vi "FSM.vi"() -> ()   [LabVIEW 2015]
uses:
  states.ctl
  globals.vi
  <vilib>/Utility/file.llb/Read Delimited Spreadsheet (DBL).vi
  read_file.vi
  output_byte.vi
panel:
  out "Progress":dbl(slide) scale=0.0..100.0
  out "Angle accuracy":dbl
  out "Current shoulder angle":dbl
  out "Current elbow angle":dbl
  in  "Stop":bool
  out "Desired shoulder Angle":dbl
  out "Desired elbow Angle":dbl
  out "Number of rows":dbl
  out "Row number":dbl
  in  "Start Button":bool
  out "State to Recover from":T1
  out "Current State":T1
  in  "Pause":bool
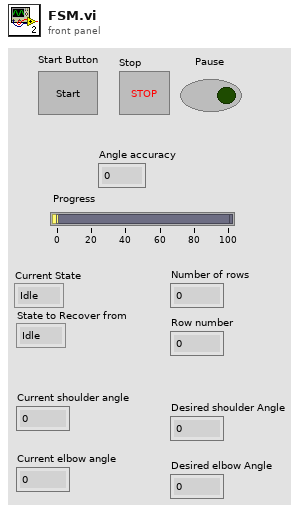
[diagram p1: front panel]
types:
  T1 = typedef "states.ctl" = enum16{"Idle", "Pause", "Next Contour", "Aligning", "Lowering Pen", "Drawing", "Next Point", "Lifting Pen", "Stop", "Put Away"}
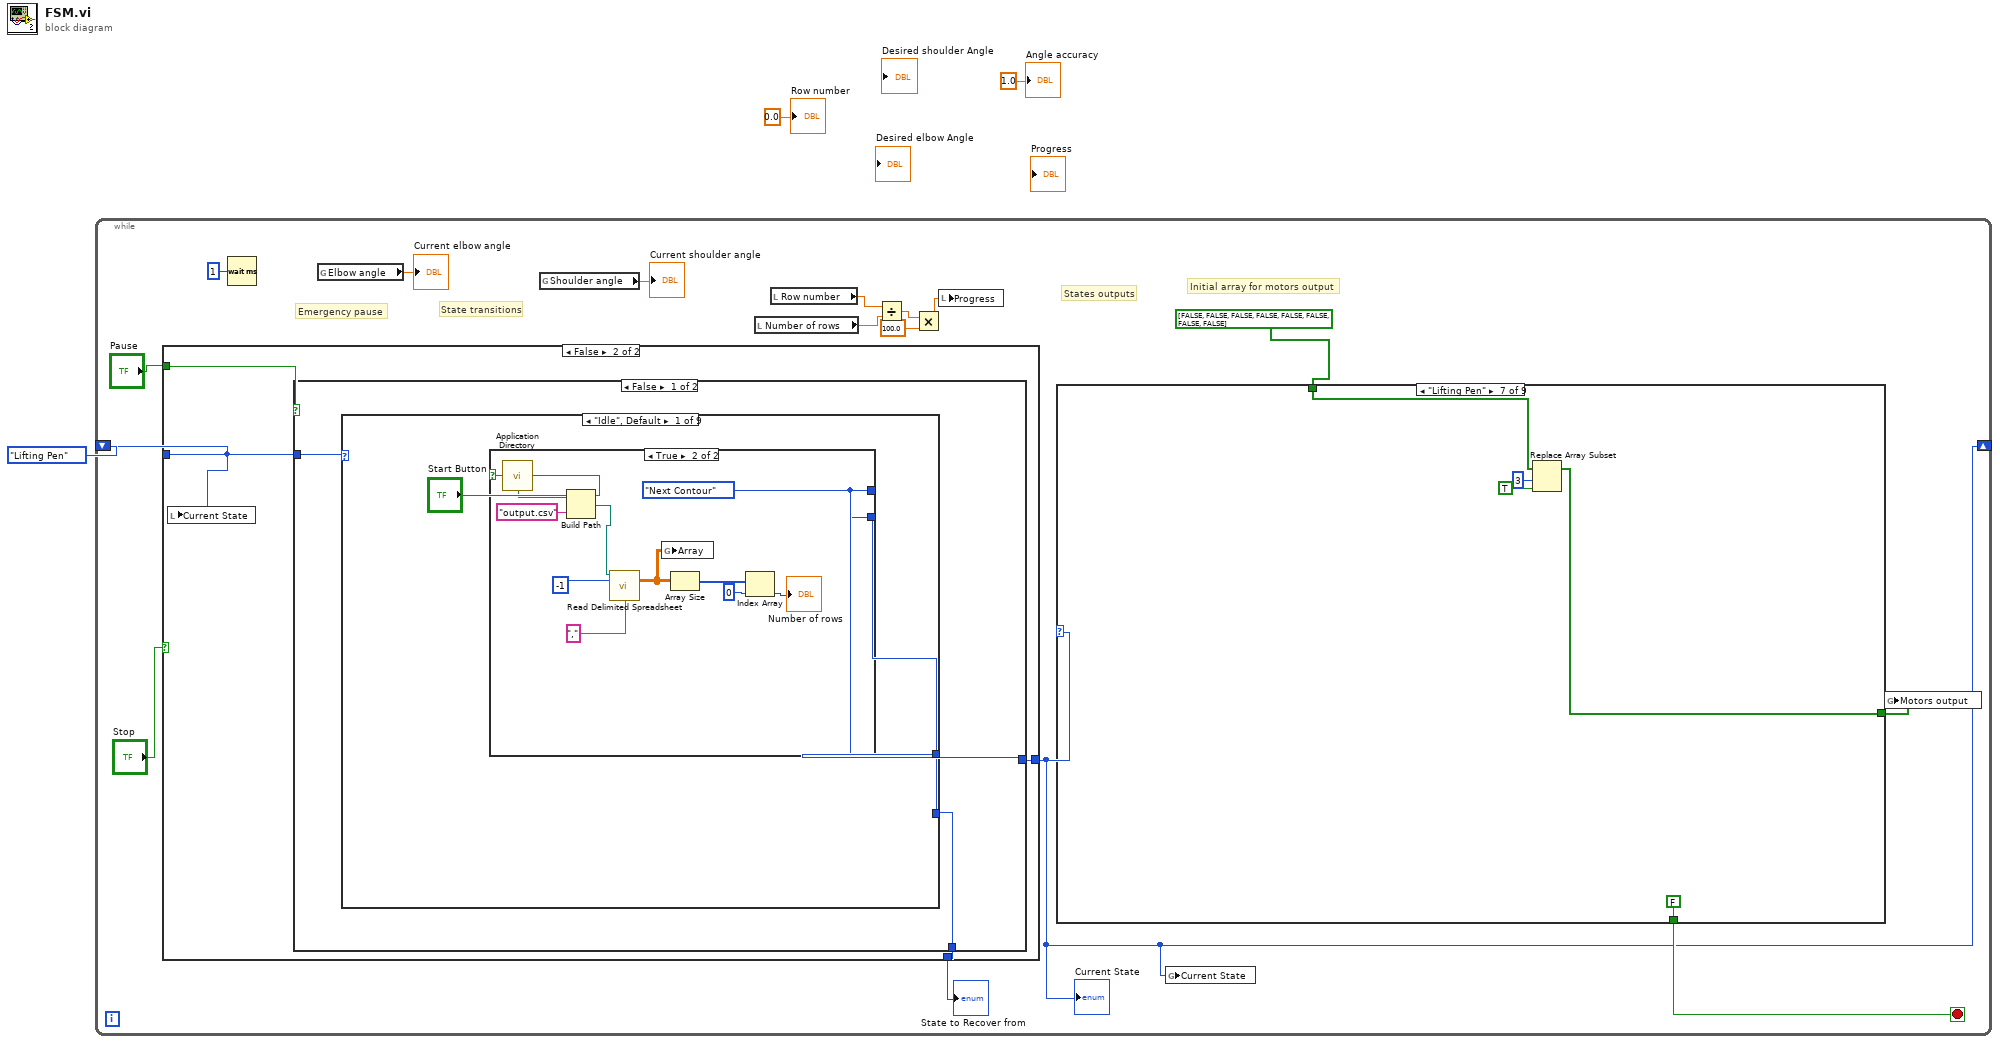
[diagram p0: block diagram]
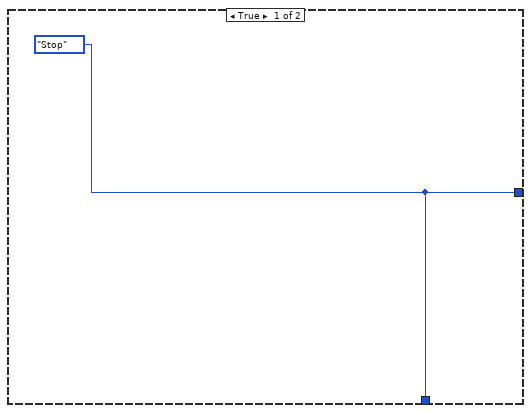
[diagram p2: hidden frame]
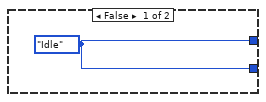
[diagram p3: hidden frame]
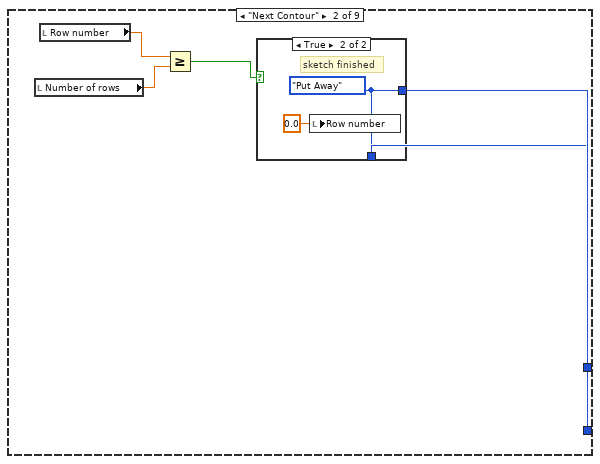
[diagram p4: hidden frame]
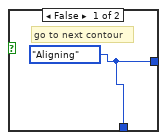
[diagram p5: hidden frame]
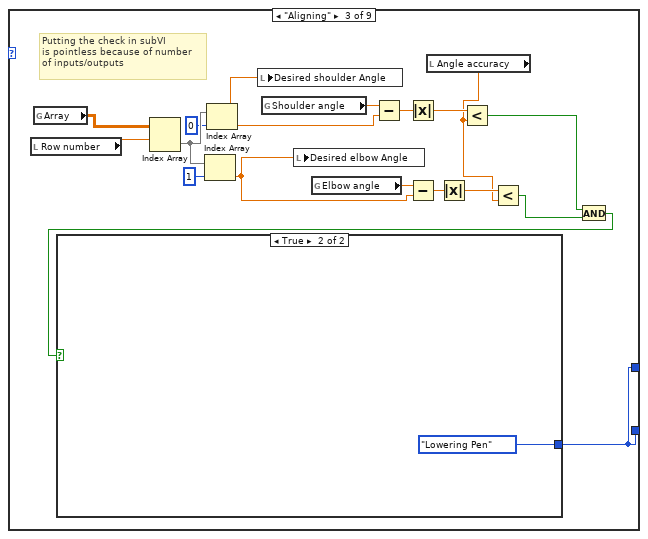
[diagram p6: hidden frame]
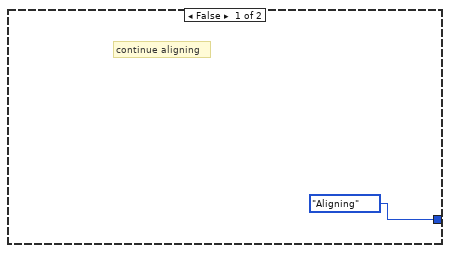
[diagram p7: hidden frame]
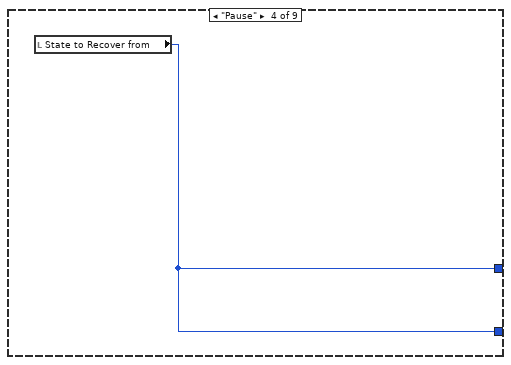
[diagram p8: hidden frame]
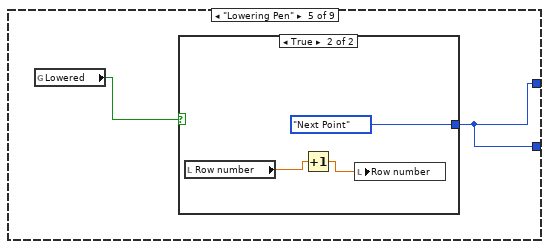
[diagram p9: hidden frame]
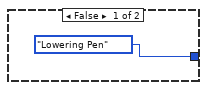
[diagram p10: hidden frame]
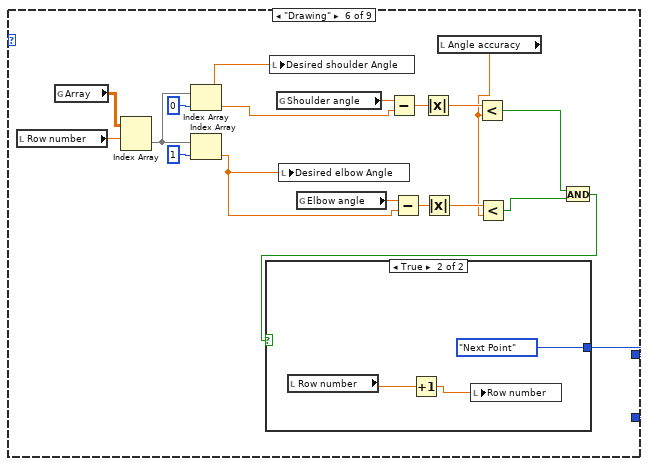
[diagram p11: hidden frame]
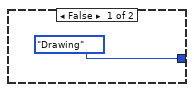
[diagram p12: hidden frame]
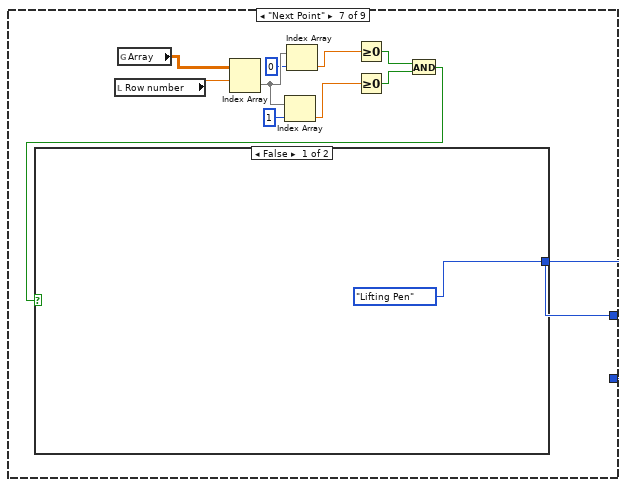
[diagram p13: hidden frame]
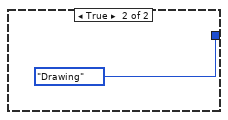
[diagram p14: hidden frame]
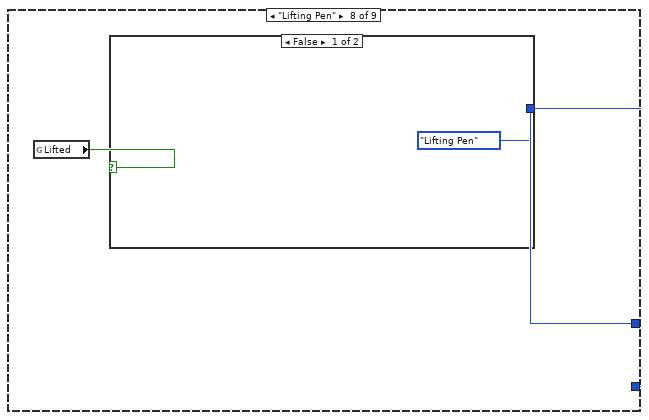
[diagram p15: hidden frame]
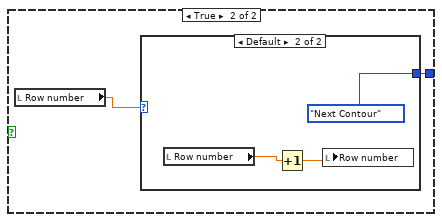
[diagram p16: hidden frame]
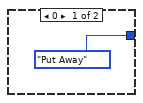
[diagram p17: hidden frame]
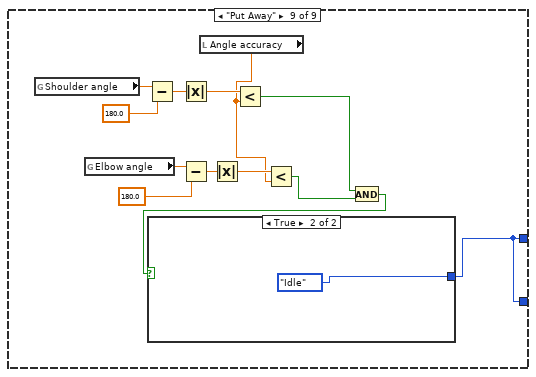
[diagram p18: hidden frame]
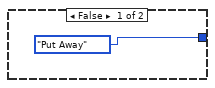
[diagram p19: hidden frame]
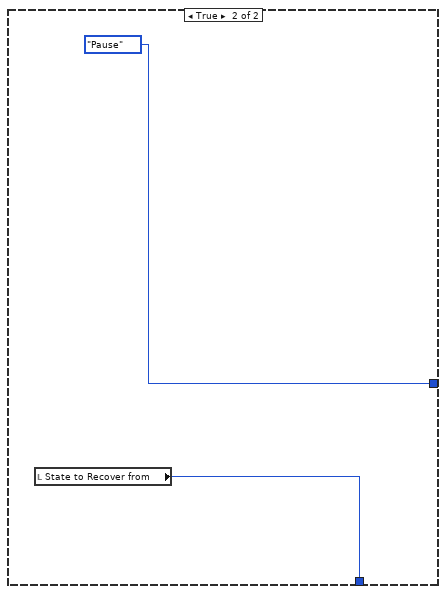
[diagram p20: hidden frame]
diagram:
  n1 = while {
    shift-right: [w4] -> _
    shift-left: states."Lifting Pen" ("State") -> [w18]
    stop <- w5 stop-if-true
    # "Initial array for motors output"
    # "States outputs"
    # "State transitions"
    # "Emergency pause"
    n2 = case shown="False" "Stop" {
      tunnel: "Pause" -> [_ w24]
      tunnel: w18 -> [_ w23]
      tunnel: [w20 w22] -> w14
      tunnel: [w20 w21] -> w4
      frame True {
        w20 = states."Stop" ("State")
      }
      frame False {
        n3 = local write "Current State"(w23) -> ()
        n4 = case shown="False" w24 {
          tunnel: w23 -> [w27 _]
          tunnel: [w26 states."Pause" ("State")] -> w21
          tunnel: [w25 w136] -> w22
          frame False {
            n5 = case shown="\"Idle\", Default" w27 {
              tunnel: [w29 w46 w54 w70 w72 w80 w100 w113 w121] -> w26
              tunnel: [w28 w45 w54 w70 w72 w80 w100 w113 w121] -> w25
              frame "Idle", Default {
                n6 = case shown="True" "Start Button" {
                  tunnel: [w31 w41] -> w29
                  tunnel: [w31 w41] -> w28
                  frame False {
                    w31 = states."Idle" ("State")
                  }
                  frame True {
                    w41 = states."Next Contour" ("State")
                    n7 = call <vilib>:"Application Directory.vi"() -> ("Application Directory"=w33:path)
                    n8 = Build Path(base path=w33, name or relative path="output.csv") -> (appended path=w32:path)
                    n9 = call-poly <vilib>:"Read Delimited Spreadsheet.vi"("file path (dialog if empty)"=w32, "number of rows (all:-1)"=-1, "delimiter (\\t)"="," ("delimiter (\\t)")) -> ("all rows"=w40:dbl[][])  [unwired: 7 in, 5 out]
                    n10 = global write "read_file.vi" "Array"(w40) -> ()
                    n11 = Array Size(array=w40) -> (size(s)=w36:i32[])
                    n12 = Index Array(array=w36, index=0) -> (element=→"Number of rows":i32)
                  }
                }
              }
              frame "Next Contour" {
                n13 = local read "Number of rows"() -> (w43:dbl)
                n14 = local read "Row number"() -> (w44:dbl)
                n15 = Greater Or Equal?(x=w44, y=w43) -> (x >= y?=w42:bool)
                n16 = case shown="True" w42 {
                  tunnel: [w47 w49] -> w46
                  tunnel: [w47 w49] -> w45
                  frame False {
                    w47 = states."Aligning" ("State")
                    # "go to next contour"
                  }
                  frame True {
                    w49 = states."Put Away" ("State")
                    # "sketch finished"
                    n17 = local write "Row number"(0.0 ("Row number")) -> ()
                  }
                }
              }
              frame "Aligning" {
                # "Putting the check in subVI\nis pointless because of number\nof inputs/outputs"
                n18 = local read "Row number"() -> (w66:dbl)
                n19 = global read "read_file.vi" "Array"() -> (w67:dbl[][])
                n20 = Index Array(array=w67, index (row)=w66) -> (element=w65:dbl[])  [unwired: 1 in]
                n21 = Index Array(array=w65, index=1) -> (element=w57:dbl)
                n22 = Index Array(array=w65, index=0) -> (element=w58:dbl)
                n23 = local write "Desired shoulder Angle"(w58) -> ()
                n24 = global read "globals.vi" "Shoulder angle"() -> (w53:dbl)
                n25 = local write "Desired elbow Angle"(w57) -> ()
                n26 = global read "globals.vi" "Elbow angle"() -> (w52:dbl)
                n27 = Subtract(x=w53, y=w58) -> (x-y=w62:dbl)
                n28 = Absolute Value(x=w62) -> (abs(x)=w61:dbl)
                n29 = Subtract(x=w52, y=w57) -> (x-y=w60:dbl)
                n30 = local read "Angle accuracy"() -> (w50:dbl)
                n31 = Absolute Value(x=w60) -> (abs(x)=w59:dbl)
                n32 = Less?(x=w61, y=w50) -> (x < y?=w56:bool)
                n33 = Less?(x=w59, y=w50) -> (x < y?=w55:bool)
                n34 = And(x=w56, y=w55) -> (x .and. y?=w51:bool)
                n35 = case shown="True" w51 {
                  tunnel: [states."Aligning" ("State") states."Lowering Pen" ("State")] -> w54
                  frame False {
                    # "continue aligning"
                  }
                  frame True {
                  }
                }
              }
              frame "Pause" {
                n36 = local read "State to Recover from"() -> (w70:T1)
              }
              frame "Lowering Pen" {
                n37 = global read "globals.vi" "Lowered"() -> (w71:bool)
                n38 = case shown="True" w71 {
                  tunnel: [states."Lowering Pen" ("State") states."Next Point" ("State")] -> w72
                  frame False {
                  }
                  frame True {
                    n39 = local read "Row number"() -> (w74:dbl)
                    n40 = Increment(x=w74) -> (x+1=w75:dbl)
                    n41 = local write "Row number"(w75) -> ()
                  }
                }
              }
              frame "Drawing" {
                n42 = local read "Row number"() -> (w81:dbl)
                n43 = global read "read_file.vi" "Array"() -> (w94:dbl[][])
                n44 = Index Array(array=w94, index (row)=w81) -> (element=w93:dbl[])  [unwired: 1 in]
                n45 = Index Array(array=w93, index=0) -> (element=w79:dbl)
                n46 = Index Array(array=w93, index=1) -> (element=w86:dbl)
                n47 = local write "Desired shoulder Angle"(w79) -> ()
                n48 = global read "globals.vi" "Shoulder angle"() -> (w83:dbl)
                n49 = local write "Desired elbow Angle"(w86) -> ()
                n50 = global read "globals.vi" "Elbow angle"() -> (w82:dbl)
                n51 = Subtract(x=w83, y=w79) -> (x-y=w90:dbl)
                n52 = Subtract(x=w82, y=w86) -> (x-y=w88:dbl)
                n53 = Absolute Value(x=w90) -> (abs(x)=w89:dbl)
                n54 = Absolute Value(x=w88) -> (abs(x)=w87:dbl)
                n55 = local read "Angle accuracy"() -> (w77:dbl)
                n56 = Less?(x=w89, y=w77) -> (x < y?=w85:bool)
                n57 = Less?(x=w87, y=w77) -> (x < y?=w84:bool)
                n58 = And(x=w85, y=w84) -> (x .and. y?=w78:bool)
                n59 = case shown="True" w78 {
                  tunnel: [states."Drawing" ("State") states."Next Point" ("State")] -> w80
                  frame False {
                  }
                  frame True {
                    n60 = local read "Row number"() -> (w97:dbl)
                    n61 = Increment(x=w97) -> (x+1=w96:dbl)
                    n62 = local write "Row number"(w96) -> ()
                  }
                }
              }
              frame "Next Point" {
                n63 = local read "Row number"() -> (w108:dbl)
                n64 = global read "read_file.vi" "Array"() -> (w109:dbl[][])
                n65 = Index Array(array=w109, index (row)=w108) -> (element=w107:dbl[])  [unwired: 1 in]
                n66 = Index Array(array=w107, index=1) -> (element=w103:dbl)
                n67 = Index Array(array=w107, index=0) -> (element=w104:dbl)
                n68 = Greater Or Equal To 0?(x=w104) -> (x >= 0?=w102:bool)
                n69 = Greater Or Equal To 0?(x=w103) -> (x >= 0?=w101:bool)
                n70 = And(x=w102, y=w101) -> (x .and. y?=w99:bool)
                n71 = case shown="False" w99 {
                  tunnel: [states."Lifting Pen" ("State") states."Drawing" ("State")] -> w100
                  frame False {
                  }
                  frame True {
                  }
                }
              }
              frame "Lifting Pen" {
                n72 = global read "globals.vi" "Lifted"() -> (w112:bool)
                n73 = case shown="False" w112 {
                  tunnel: [states."Lifting Pen" ("State") w116] -> w113
                  frame False {
                  }
                  frame True {
                    n74 = local read "Row number"() -> (w115:dbl)
                    n75 = case shown="Default" w115 {
                      tunnel: [states."Put Away" ("State") states."Next Contour" ("State")] -> w116
                      frame 0 {
                      }
                      frame Default {
                        n76 = local read "Row number"() -> (w119:dbl)
                        n77 = Increment(x=w119) -> (x+1=w118:dbl)
                        n78 = local write "Row number"(w118) -> ()
                      }
                    }
                  }
                }
              }
              frame "Put Away" {
                n79 = global read "globals.vi" "Shoulder angle"() -> (w127:dbl)
                n80 = global read "globals.vi" "Elbow angle"() -> (w126:dbl)
                n81 = Subtract(x=w127, y=180.0) -> (x-y=w133:dbl)
                n82 = Absolute Value(x=w133) -> (abs(x)=w132:dbl)
                n83 = Subtract(x=w126, y=180.0) -> (x-y=w131:dbl)
                n84 = local read "Angle accuracy"() -> (w125:dbl)
                n85 = Absolute Value(x=w131) -> (abs(x)=w130:dbl)
                n86 = Less?(x=w132, y=w125) -> (x < y?=w129:bool)
                n87 = Less?(x=w130, y=w125) -> (x < y?=w128:bool)
                n88 = And(x=w129, y=w128) -> (x .and. y?=w122:bool)
                n89 = case shown="True" w122 {
                  tunnel: [states."Put Away" ("State") states."Idle" ("State")] -> w121
                  frame False {
                  }
                  frame True {
                  }
                }
              }
            }
          }
          frame True {
            n90 = local read "State to Recover from"() -> (w136:T1)
          }
        }
      }
    }
    "Current State" <- w4
    "State to Recover from" <- w14
    n91 = Wait (ms)(milliseconds to wait=u32 1 ("millisecond multiple")) -> ()  [unwired: 1 out]
    n92 = global read "globals.vi" "Elbow angle"() -> (→"Current elbow angle":dbl)
    n93 = global read "globals.vi" "Shoulder angle"() -> (→"Current shoulder angle":dbl)
    n94 = local read "Number of rows"() -> (w10:dbl)
    n95 = local read "Row number"() -> (w11:dbl)
    n96 = Divide(x=w11, y=w10) -> (x/y=w9:dbl)
    n97 = Multiply(x=w9, y=100.0) -> (x*y=w7:dbl)
    n98 = local write "Progress"(w7) -> ()
    n99 = case shown="\"Lifting Pen\"" w4 {
      tunnel: bool[] [FALSE, FALSE, FALSE, FALSE, FALSE, FALSE, FALSE, FALSE] -> [w139 w141 w143 w146 w167 w198 w201 w205 w209]
      tunnel: [w139 w141 w143 w145 w166 w198 w200 w205 w206] -> w12
      tunnel: [FALSE FALSE FALSE FALSE FALSE FALSE FALSE TRUE FALSE] -> w5
      frame "Idle", Default {
      }
      frame "Pause" {
      }
      frame "Next Contour" {
      }
      frame "Lowering Pen" {
        n100 = Replace Array Subset(array=w146, new element=TRUE ("new element/subarray"), index=2) -> (w145:bool[])
      }
      frame "Aligning", "Drawing" {
        n101 = local read "Row number"() -> (w162:dbl)
        n102 = global read "read_file.vi" "Array"() -> (w161:dbl[][])
        n103 = global read "globals.vi" "Shoulder angle"() -> (w160:dbl)
        n104 = global read "globals.vi" "Elbow angle"() -> (w156:dbl)
        n105 = Index Array(array=w161, index (row)=w162) -> (element=w163:dbl[])  [unwired: 1 in]
        n106 = Index Array(array=w163, index=1) -> (element=w153:dbl)
        n107 = local write "Desired elbow Angle"(w153) -> ()
        n108 = Index Array(array=w163, index=0) -> (element=w157:dbl)
        n109 = local write "Desired shoulder Angle"(w157) -> ()
        n110 = local read "Angle accuracy"() -> (w150:dbl)
        n111 = Subtract(x=w160, y=w157) -> (x-y=w158:dbl)
        n112 = Subtract(x=w156, y=w153) -> (x-y=w154:dbl)
        n113 = Absolute Value(x=w158) -> (abs(x)=w159:dbl)
        n114 = Absolute Value(x=w154) -> (abs(x)=w155:dbl)
        n115 = Less?(x=w159, y=w150) -> (x < y?=w152:bool)
        n116 = Less?(x=w155, y=w150) -> (x < y?=w151:bool)
        n117 = case shown="False" w151 {
          tunnel: [w184 w196] -> w168
          tunnel: w167 -> [w183 w196]
          frame False {
            n118 = local read "Desired elbow Angle"() -> (w187:dbl)
            n119 = global read "globals.vi" "Elbow angle"() -> (w185:dbl)
            n120 = Greater?(x=w185, y=w187) -> (0:w186:bool)
            n121 = case shown="False" w186 {
              tunnel: [w189 w193] -> w184
              tunnel: w183 -> [w188 w192]
              frame False {
                n122 = Replace Array Subset(array=w188, new element=TRUE ("new element/subarray"), index=5) -> (w189:bool[])
              }
              frame True {
                n123 = Replace Array Subset(array=w192, new element=TRUE ("new element/subarray"), index=4) -> (w193:bool[])
              }
            }
          }
          frame True {
          }
        }
        n124 = case shown="False" w152 {
          tunnel: [w171 w182] -> w166
          tunnel: w168 -> [w169 w182]
          frame False {
            n125 = local read "Desired shoulder Angle"() -> (w170:dbl)
            n126 = global read "globals.vi" "Shoulder angle"() -> (w172:dbl)
            n127 = Greater?(x=w172, y=w170) -> (0:w173:bool)
            n128 = case shown="False" w173 {
              tunnel: [w175 w179] -> w171
              tunnel: w169 -> [w174 w178]
              frame False {
                n129 = Replace Array Subset(array=w174, new element=TRUE ("new element/subarray"), index=7) -> (w175:bool[])
              }
              frame True {
                n130 = Replace Array Subset(array=w178, new element=TRUE ("new element/subarray"), index=6) -> (w179:bool[])
              }
            }
          }
          frame True {
          }
        }
      }
      frame "Next Point" {
      }
      frame "Lifting Pen" {
        n131 = Replace Array Subset(array=w201, new element=TRUE ("new element/subarray"), index=3) -> (w200:bool[])
      }
      frame "Stop" {
      }
      frame "Put Away" {
        n132 = global read "globals.vi" "Shoulder angle"() -> (w218:dbl)
        n133 = global read "globals.vi" "Elbow angle"() -> (w215:dbl)
        n134 = local read "Angle accuracy"() -> (w210:dbl)
        n135 = Subtract(x=w218, y=180.0) -> (x-y=w216:dbl)
        n136 = Subtract(x=w215, y=180.0) -> (x-y=w213:dbl)
        n137 = Absolute Value(x=w216) -> (abs(x)=w217:dbl)
        n138 = Absolute Value(x=w213) -> (abs(x)=w214:dbl)
        n139 = Less?(x=w217, y=w210) -> (x < y?=w212:bool)
        n140 = Less?(x=w214, y=w210) -> (x < y?=w211:bool)
        n141 = case shown="False" w211 {
          tunnel: [w237 w248] -> w219
          tunnel: w209 -> [w236 w248]
          frame False {
            n142 = global read "globals.vi" "Elbow angle"() -> (w238:dbl)
            n143 = Greater?(x=w238, y=180.0) -> (0:w239:bool)
            n144 = case shown="False" w239 {
              tunnel: [w241 w245] -> w237
              tunnel: w236 -> [w240 w244]
              frame False {
                n145 = Replace Array Subset(array=w240, new element=TRUE ("new element/subarray"), index=5) -> (w241:bool[])
              }
              frame True {
                n146 = Replace Array Subset(array=w244, new element=TRUE ("new element/subarray"), index=4) -> (w245:bool[])
              }
            }
          }
          frame True {
          }
        }
        n147 = case shown="False" w212 {
          tunnel: [w223 w234] -> w206
          tunnel: w219 -> [w222 w234]
          frame False {
            n148 = global read "globals.vi" "Shoulder angle"() -> (w224:dbl)
            n149 = Greater?(x=w224, y=180.0) -> (0:w225:bool)
            n150 = case shown="False" w225 {
              tunnel: [w227 w231] -> w223
              tunnel: w222 -> [w226 w230]
              frame False {
                n151 = Replace Array Subset(array=w226, new element=TRUE ("new element/subarray"), index=7) -> (w227:bool[])
              }
              frame True {
                n152 = Replace Array Subset(array=w230, new element=TRUE ("new element/subarray"), index=6) -> (w231:bool[])
              }
            }
          }
          frame True {
          }
        }
      }
    }
    n153 = global write "output_byte.vi" "Current State"(w4) -> ()
    n154 = global write "output_byte.vi" "Motors output"(w12) -> ()
  }
  "Row number" <- 0.0 ("Row number")
  "Angle accuracy" <- 1.0 ("Angle accuracy")
